vi "Rotary Table.vi"(10 "VISA resource name":refnum<visa-resource-name>="COM2", 11 "string to write":string) -> (2 "read buffer":string, 3 "bytes read":u32)   [LabVIEW 2023]
uses:
  <vilib>/Instr/_visa.llb/VISA Configure Serial Port (Instr).vi
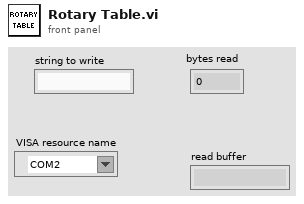
[diagram p1: front panel]
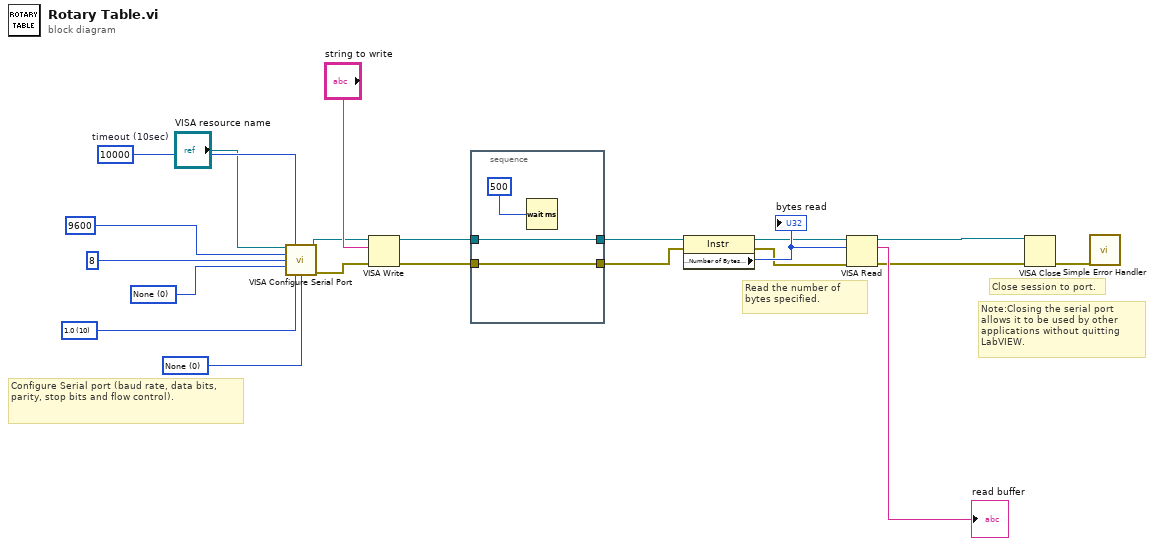
[diagram p0: block diagram]
diagram:
  w11 = u16 0 items=["None"=0, "XON/XOFF"=1, "RTS/CTS"=2, "DTR/DSR"=4] ("flow control")
  w10 = u16 10 items=["1.0"=10, "1.5"=15, "2.0"=20] ("stop bits")
  w8 = u16 0 items=["None", "Odd", "Even", "Mark", "Space"] ("parity")
  w9 = u32 10000  # timeout (10sec)
  # "Read the number of bytes specified."
  # "Note:Closing the serial port allows it to be used by other applications without quitting LabVIEW."
  # "Configure Serial port (baud rate, data bits, parity, stop bits and flow control)."
  # "Close session to port."
  n1 = call-poly "VISA Configure Serial Port"("VISA resource name"="VISA resource name", "timeout (10sec)"=w9, "baud rate (9600)"=u32 9600 ("baud rate"), "data bits (8)"=u16 8 ("data bits"), "parity (0:none)"=w8, "stop bits (10: 1 bit)"=w10, "flow control (0:none)"=w11) -> ("VISA resource name out"=w4:refnum<visa-resource-name>, "error out"=w3:errorcluster)  [unwired: 2 in, 5 out]
  n2 = VISA Write(VISA resource name=w4, write buffer="string to write", error in (no error)=w3) -> (VISA resource name out=w15:refnum<visa-resource-name>, error out=w13:errorcluster)  [unwired: 1 out]
  n3 = stacked-sequence {
    tunnel: w13 -> [w24]
    tunnel: [w24] -> w14
    tunnel: w15 -> [w23]
    tunnel: [w23] -> w16
    frame #0 {
      n4 = Wait (ms)(milliseconds to wait=u32 500 ("delay before read (ms)")) -> ()  [unwired: 1 out]
    }
  }
  n5 = property class="Instr"(reference=w16, error in=w14) -> (reference out=w18:refnum<visa-resource-name>, error out=w19:errorcluster, "Serial Settings:Number of Bytes at Serial Port"=w21:u32)
  "bytes read" <- w21
  n6 = VISA Read(VISA resource name=w18, byte count=w21, error in (no error)=w19) -> (VISA resource name out=w6:refnum<visa-resource-name>, read buffer=→"read buffer":string, error out=w5:errorcluster)  [unwired: 1 out]
  n7 = VISA Close(VISA resource name=w6, error in (no error)=w5) -> (error out=w7:errorcluster)
  n8 = call <vilib>:"Simple Error Handler.vi"("error in (no error)"=w7) -> ()  [unwired: 1 in, 8 out]
